vi "Manipulator Limits.vi"(8 "error in (no error)":errorcluster, 11 "VISA resource in":refnum<visa-resource-name>="COM1") -> (0 "error out":errorcluster, 2 "Boolean":bool=TRUE, 3 "VISA resource out":refnum<visa-resource-name>)   [LabVIEW 2012, in "Scientifica Manipulator Daemon.lvlib"]
uses:
  Scientifica Manipulator Daemon.lvlib
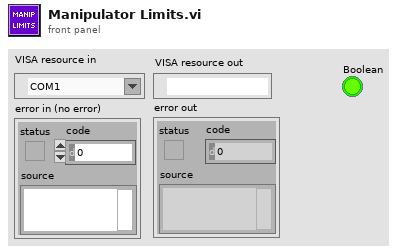
[diagram p1: front panel]
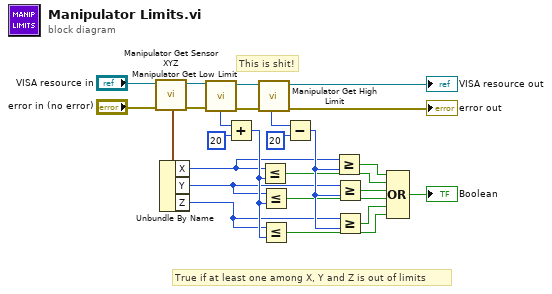
[diagram p0: block diagram]
diagram:
  # "This is shit!"
  # "True if at least one among X, Y and Z is out of limits"
  n1 = call "Manipulator Get Sensor XYZ.vi"("error in (no error)"="error in (no error)", "VISA resource in"="VISA resource in") -> ("error out"=w21:errorcluster, "output cluster"=w25:cluster{"X":i32, "Y":i32, "Z":i32, "A":i32}, "VISA resource out"=w22:refnum<visa-resource-name>)  [unwired: 7 in]
  n2 = Unbundle By Name(w25) -> ("X"=w3:i32, "Y"=w12:i32, "Z"=w11:i32)
  n3 = call "Manipulator Get Low Limit.vi"("error in (no error)"=w21, "VISA resource in"=w22) -> ("error out"=w23:errorcluster, "Low Limit"=w16:i32, "VISA resource out"=w24:refnum<visa-resource-name>)  [unwired: 7 in]
  n4 = Add(x=w16, y=20) -> (x+y=w13:i32)
  n5 = call "Manipulator Get High Limit.vi"("error in (no error)"=w23, "VISA resource in"=w24) -> ("error out"=→"error out":errorcluster, "High Limit"=w17:i32, "VISA resource out"=→"VISA resource out":refnum<visa-resource-name>)  [unwired: 7 in]
  n6 = Less Or Equal?(x=w3, y=w13) -> (x <= y?=w9:bool)
  n7 = Less Or Equal?(x=w12, y=w13) -> (x <= y?=w7:bool)
  n8 = Less Or Equal?(x=w11, y=w13) -> (x <= y?=w5:bool)
  n9 = Subtract(x=w17, y=20) -> (x-y=w14:i32)
  n10 = Greater Or Equal?(x=w3, y=w14) -> (x >= y?=w10:bool)
  n11 = Greater Or Equal?(x=w12, y=w14) -> (x >= y?=w8:bool)
  n12 = Greater Or Equal?(x=w11, y=w14) -> (x >= y?=w6:bool)
  n13 = Compound Arithmetic op=OR(w10, w9, w8, w7, w6, w5) -> (→"Boolean":bool)
